vi "SQLEndTran.vi"(4 "error in (no error)":errorcluster, 5 "CompletionType":bool, 6 "HandleType":T1(ring)=enum."SQL_HANDLE_ENV", 7 "InputHandle":i32) -> (0 "error out":errorcluster)   [LabVIEW 2011]
doc: "Valide ou invalide la transaction spécifiée par le lien ODBC"
uses:
  Odbc32.dll
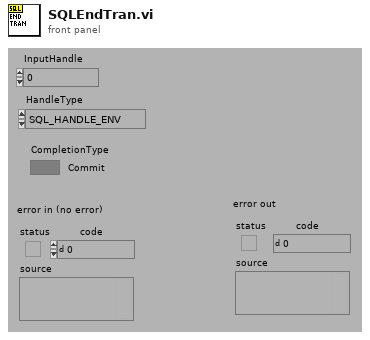
[diagram p1: front panel]
types:
  T1 = enum16{"NOPE", "SQL_HANDLE_ENV", "SQL_HANDLE_DBC", "SQL_HANDLE_STMT", "SQL_HANDLE_DESC"}
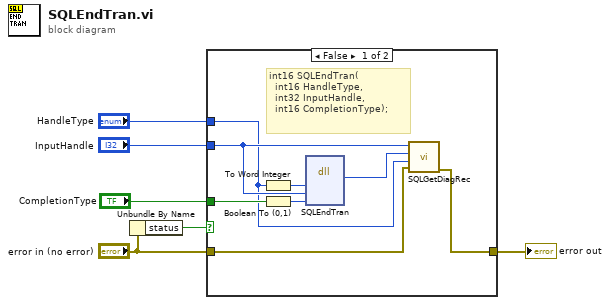
[diagram p0: block diagram]
diagram:
  n1 = Unbundle By Name("error in (no error)") -> ("status"=w3:bool)
  n2 = case shown="False" w3 {
    tunnel: "CompletionType" -> [w14 _]
    tunnel: "HandleType" -> [w7 _]
    tunnel: "InputHandle" -> [w10 _]
    tunnel: "error in (no error)" -> [w9 w15]
    tunnel: [w8 w15] -> w1
    frame False {
      # "int16 SQLEndTran(\n  int16 HandleType, \n  int32 InputHandle, \n  int16 CompletionType);"
      n3 = To Word Integer(number=w7) -> (16bit integer=w12:i16)
      n4 = Boolean To (0,1)(Boolean=w14) -> (0, 1=w13:i16)
      n5 = dll-call lib="Odbc32.dll" fn="SQLEndTran"("HandleType"=w12, "InputHandle"=w10, "CompletionType"=w13) -> (w11:i16)  [unwired: 6 in, 2 out]
      n6 = call "SQLGetDiagRec.vi"("error in (no error)"=w9, "HandleType"=w7, "Status (SQL_SUCCESS=0)"=w11, "Input Handle"=w10) -> ("error out"=w8:errorcluster)  [unwired: 3 out]
    }
    frame True {
    }
  }
  "error out" <- w1
